vi "Data Read Control.vi"(7 "Pixel time up":bool, 8 "DRAM pack index out in":T1, 9 "input valid?":bool, 10 "DRAM pack index out":T1) -> (3 "output valid":bool)   [LabVIEW 2015]
uses:
  DRAM data index.ctl
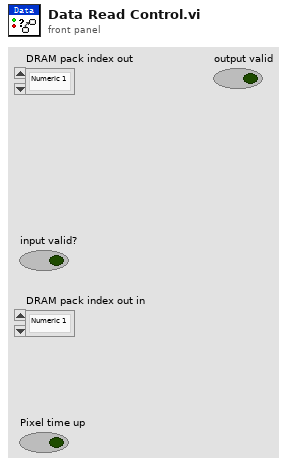
[diagram p1: front panel]
types:
  T1 = typedef "DRAM data index.ctl" = enum16{"Numeric 1", "Numeric 2", "Numeric 3", "Numeric 4", "Numeric 5", "Numeric 6", "Numeric 7", "Numeric 8", "Numeric 9", "Numeric 10", "Numeric 11", "Numeric 12", "Numeric 13", "Numeric 14", "Numeric 15", "Numeric 16"}
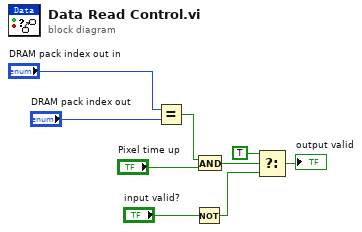
[diagram p0: block diagram]
diagram:
  n1 = Equal?(x="DRAM pack index out in", y="DRAM pack index out") -> (x = y?=w3:bool)
  n2 = Not(x="input valid?") -> (.not. x?=w5:bool)
  n3 = And(x=w3, y="Pixel time up") -> (x .and. y?=w4:bool)
  n4 = Select(t=TRUE, s=w4, f=w5) -> (s? t:f=→"output valid":bool)
